vi "HP 3458 Digitizer.vi"(1 "Ask Save Data":bool, 2 "Time Spacing":dbl=0.00025 format="%.3e", 3 "# Points":u32=4000, 4 "VISA session":refnum<visa-resource-name>) -> (0 "Measurement":dbl[](array[numeric]) format="%.5e")   [LabVIEW 2019]
doc: "This VI reads a single reading from a HP 34401 multimeter. The stop boolean is always false. If no reading is obtained a single zero is returned.\nScott Hannahs, NHMFL-FSU, April 1994"
uses:
  <vilib>/Analysis/NI_AALBase.lvlib
panel:
  out "Max variation - PPM":dbl format="%.1f"
  out "done":bool
  out "PPM Noise":dbl format="%.1f"
  out "Std. Dev":dbl format="%.3e"
  out "Ave":dbl format="%.7e"
  out "?":cluster{dbl, "Time Spacing":dbl, dbl[]}(graph)
  in  "?":i32[](array[numeric])
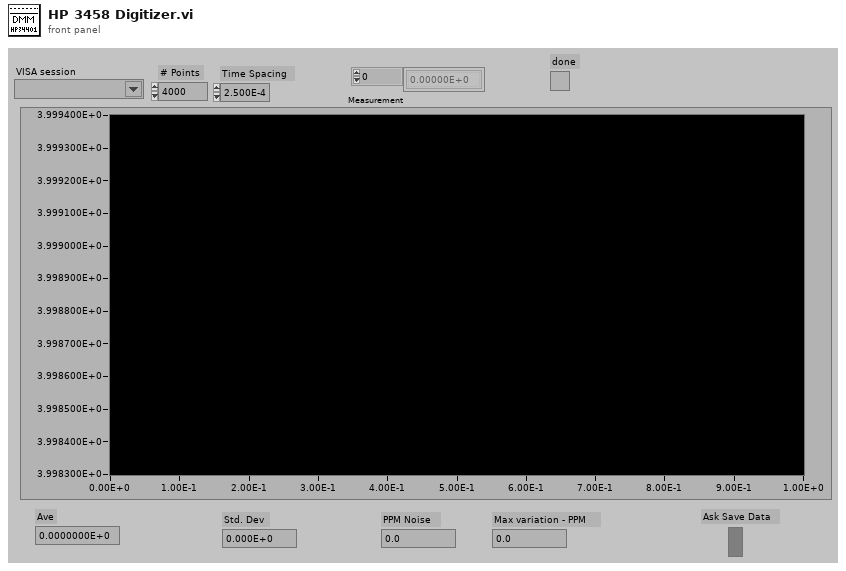
[diagram p1: front panel]
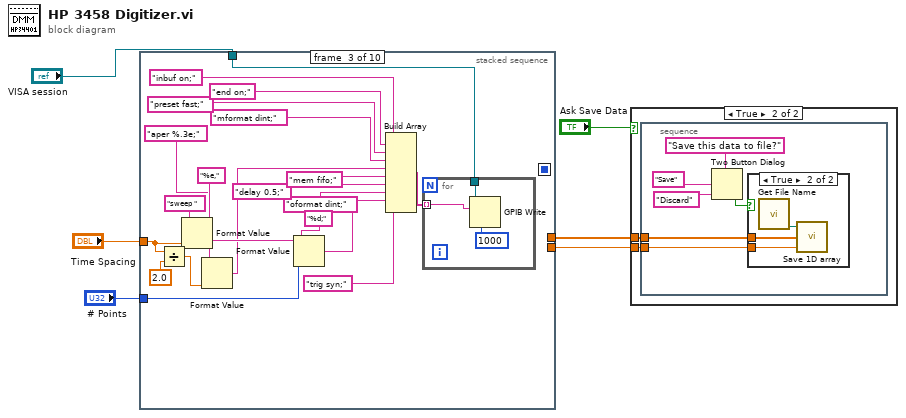
[diagram p0: block diagram]
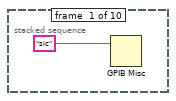
[diagram p4: hidden frame]
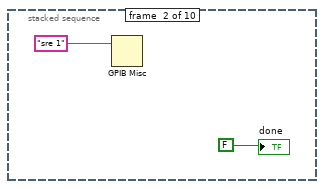
[diagram p5: hidden frame]
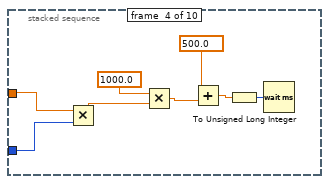
[diagram p6: hidden frame]
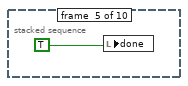
[diagram p7: hidden frame]
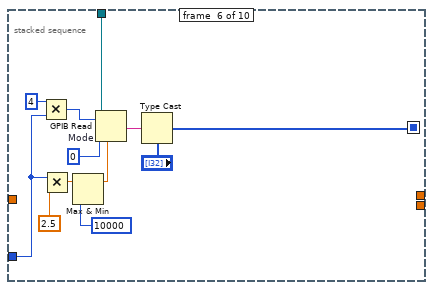
[diagram p8: hidden frame]
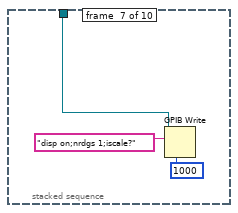
[diagram p9: hidden frame]
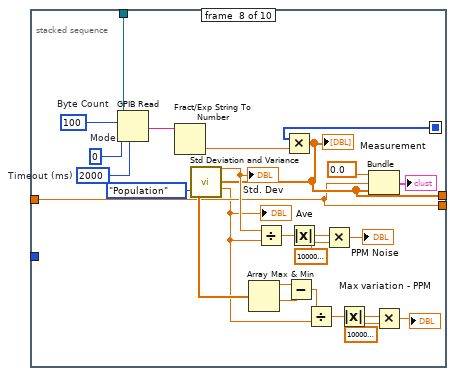
[diagram p10: hidden frame]
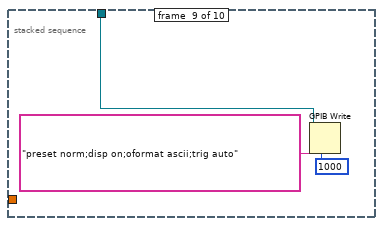
[diagram p11: hidden frame]
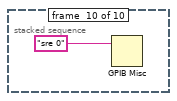
[diagram p12: hidden frame]
diagram:
  n1 = stacked-sequence {
    seq-local: [_ _ _ _ _ w51 _ _ _ _] -> [_ _ _ _ _ _ _ w78 _ _]
    tunnel: "VISA session" -> [_ _ w25 _ _ w53 w56 w79 w84 _]
    tunnel: "Time Spacing" -> [_ _ w22 w39 _ _ _ w67 _ _]
    tunnel: "# Points" -> [_ _ w26 w38 _ w46 _ _ _ _]
    tunnel: [_ _ _ _ _ _ _ w68 _ _] -> w4
    tunnel: [_ _ _ _ _ _ _ w67 _ _] -> w3
    frame #0 {
      n2 = GPIB Misc(0:"sic") -> ()  [unwired: 1 in, 3 out]
    }
    frame #1 {
      n3 = GPIB Misc(0:"sre 1") -> ()  [unwired: 1 in, 3 out]
      "done" <- FALSE
    }
    frame #2 {
      n4 = Divide(x=w22, y=2.0) -> (x/y=w20:dbl)
      n5 = Format Value(string ("")="sweep ", format string="%e,", value (0)=w22) -> (output string=w29:string)
      n6 = Format Value(format string="aper %.3e;", value (0)=w20) -> (output string=w18:string)  [unwired: 1 in]
      n7 = Format Value(string ("")=w29, format string="%d;", value (0)=w26) -> (output string=w24:string)
      n8 = Build Array("inbuf on;", "end on;", "preset fast;", "mformat dint;", w18, "mem fifo;", "delay 0.5;", "oformat dint;", w24, "trig syn;") -> (w23:string[])
      n9 = for {
        tunnel: w25 -> [w32]
        tunnel: w23 -> [w31] mode=indexing
        n10 = GPIB Write(0:w32, 1:w31, 4:u32 1000) -> ()  [unwired: 2 in, 2 out]
      }
    }
    frame #3 {
      n11 = Multiply(x=w39, y=w38) -> (x*y=w40:dbl)
      n12 = Multiply(x=1000.0, y=w40) -> (x*y=w37:dbl)
      n13 = Add(x=500.0, y=w37) -> (x+y=w35:dbl)
      n14 = To Unsigned Long Integer(number=w35) -> (unsigned 32bit integer=w36:u32)
      n15 = Wait (ms)(milliseconds to wait=w36) -> ()  [unwired: 1 out]
    }
    frame #4 {
      n16 = local write "done"(TRUE) -> ()
    }
    frame #5 {
      w54 = 0  # Mode
      n17 = Multiply(x=u32 4, y=w46) -> (x*y=w49:u32)
      n18 = Multiply(x=w46, y=2.5) -> (x*y=w44:dbl)
      n19 = Max & Min(x=w44, y=10000) -> (max(x,y)=w47:dbl)  [unwired: 1 out]
      n20 = GPIB Read(0:w53, 1:w49, 2:w54, 4:w47) -> (5:w48:string)  [unwired: 1 in, 2 out]
      n21 = Type Cast(type="?", x=w48) -> (*(type *) &x=w51:i32[])
    }
    frame #6 {
      n22 = GPIB Write(0:w56, 1:"disp on;nrdgs 1;iscale?", 4:u32 1000) -> ()  [unwired: 2 in, 2 out]
    }
    frame #7 {
      w81 = u32 2000  # Timeout (ms)
      w80 = 100  # Byte Count
      w82 = 0  # Mode
      n23 = GPIB Read(0:w79, 1:w80, 2:w82, 4:w81) -> (5:w77:string)  [unwired: 1 in, 2 out]
      n24 = Fract/Exp String To Number(string=w77) -> (number=w76:dbl)  [unwired: 3 in, 1 out]
      n25 = Multiply(x=w78, y=w76) -> (x*y=w68:dbl[])
      "Measurement" <- w68
      n26 = call <vilib>:"Std Deviation and Variance.vi"("X"=w68, "Weighting (Sample)"=enum16{"Sample", "Population"}."Population") -> ("mean"=w60:dbl, "standard deviation"=w75:dbl)  [unwired: 1 out]
      "Std. Dev" <- w75
      "Ave" <- w60
      n27 = Array Max & Min(array=w68) -> (max value=w66:dbl, min value=w65:dbl)  [unwired: 2 out]
      n28 = Divide(x=w75, y=w60) -> (x/y=w74:dbl)
      n29 = Subtract(x=w66, y=w65) -> (x-y=w61:dbl)
      n30 = Absolute Value(x=w74) -> (abs(x)=w71:dbl)
      n31 = Divide(x=w61, y=w60) -> (x/y=w62:dbl)
      n32 = Multiply(x=w71, y=1000000.0) -> (x*y=→"PPM Noise":dbl)
      n33 = Absolute Value(x=w62) -> (abs(x)=w64:dbl)
      n34 = Bundle(0.0, "Time Spacing"=w67, w68) -> (→"?":cluster{dbl, "Time Spacing":dbl, dbl[]})  [unwired: 1 in]
      n35 = Multiply(x=w64, y=1000000.0) -> (x*y=→"Max variation - PPM":dbl)
    }
    frame #8 {
      n36 = GPIB Write(0:w84, 1:"preset norm;disp on;oformat ascii;trig auto", 4:u32 1000) -> ()  [unwired: 2 in, 2 out]
    }
    frame #9 {
      n37 = GPIB Misc(0:"sre 0") -> ()  [unwired: 1 in, 3 out]
    }
  }
  n38 = case shown="True" "Ask Save Data" {
    tunnel: w4 -> [_ w88]
    tunnel: w3 -> [_ w87]
    frame False {
    }
    frame True {
      n39 = stacked-sequence {
        tunnel: w88 -> [w90]
        tunnel: w87 -> [w89]
        frame #0 {
          n40 = Two Button Dialog(message="Save this data to file?", 1:"Discard", 2:"Save") -> (T button?=w94:bool)
          n41 = case shown="True" w94 {
            tunnel: w90 -> [_ w96]
            tunnel: w89 -> [_ w95]
            frame False {
            }
            frame True {
              n42 = call "Get File Name.vi"() -> (w97:path)
              n43 = call "Save 1D array.vi"("ÆT"=w95, "Data"=w96, "File Path"=w97) -> ()
            }
          }
        }
      }
    }
  }
